vi "BatterySimulator.vi"() -> ()   [LabVIEW 2015]
panel:
  out "Waveform Graph 2":i32[](graph)
  out "Waveform Graph":dbl[](graph)
  out "exp(x)":fxp<+/-,64,32>
  out "x*y":dbl
  out "x/y":dbl
  out "Is":dbl
  out "Is  factor":dbl
  out "x-y":dbl
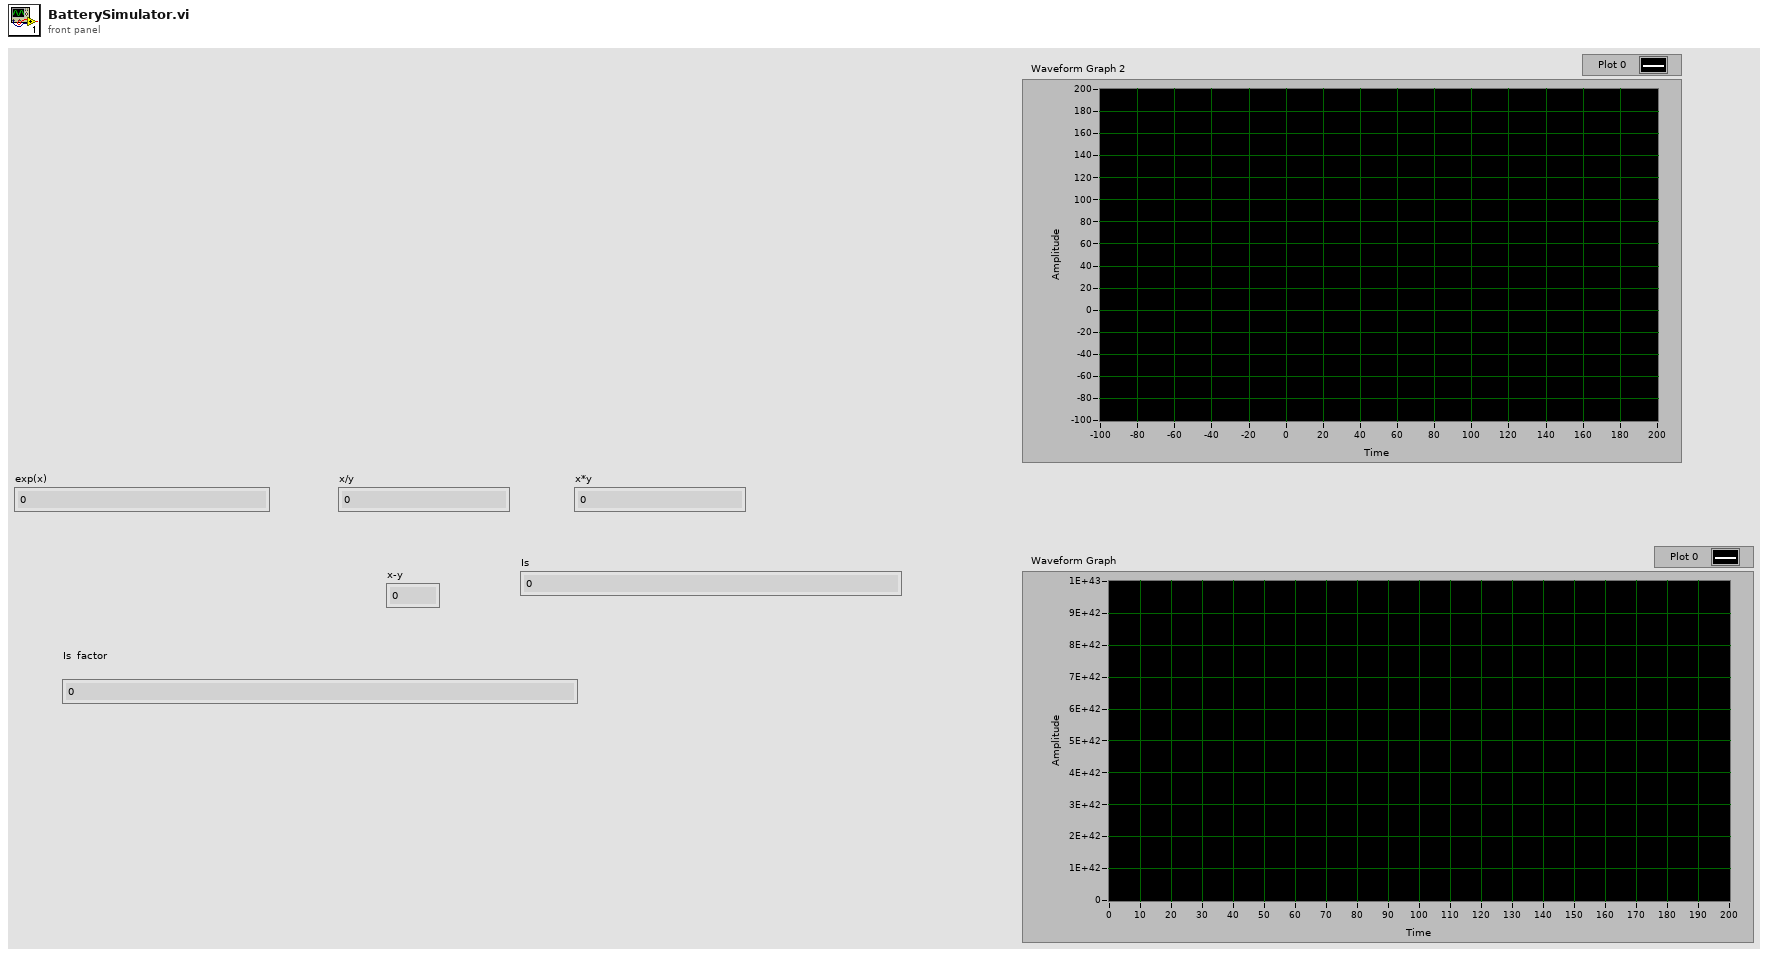
[diagram p1: front panel]
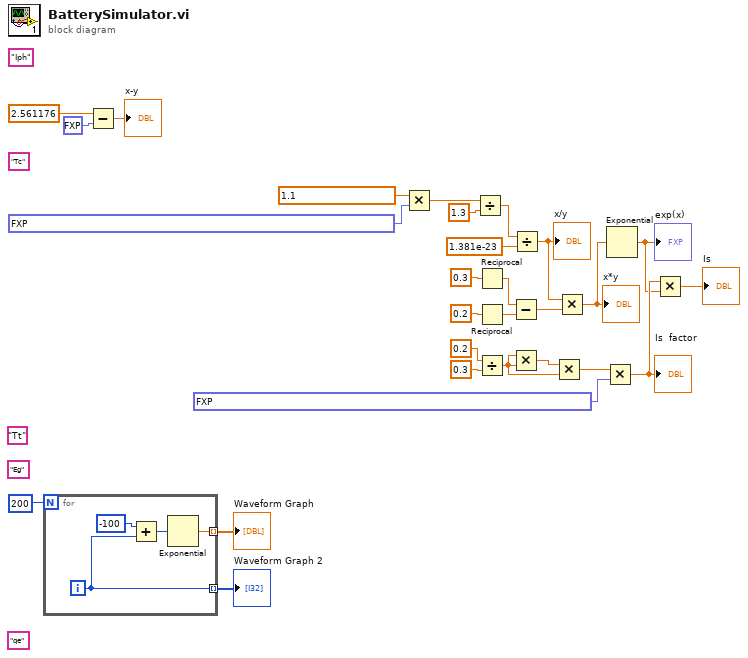
[diagram p0: block diagram]
diagram:
  (unwired) "Eg"
  (unwired) "qe"
  (unwired) "Tt"
  (unwired) "Tc"
  (unwired) "Iph"
  n1 = for {
    N: 200 -> [_]
    tunnel: [w30] -> w2 mode=indexing
    tunnel: [w29] -> w1 mode=indexing
    i -> [w29]
    n2 = Add(x=-100, y=w29) -> (x+y=w32:i32)
    n3 = Exponential(1:w32) -> (0:w30:dbl)
  }
  "Waveform Graph" <- w2
  "Waveform Graph 2" <- w1
  n4 = Subtract(x=2.561176, y=fxp<+,1,1> 0.0) -> (x-y=→"x-y":dbl)
  n5 = Multiply(x=1.1, y=fxp<+,15,-62> 1.6020172359436998e-19) -> (x*y=w14:dbl)
  n6 = Divide(x=w14, y=1.3) -> (x/y=w12:dbl)
  n7 = Reciprocal(x=0.3) -> (1/x=w8:dbl)
  n8 = Reciprocal(x=0.2) -> (1/x=w7:dbl)
  n9 = Divide(x=0.2, y=0.3) -> (x/y=w21:dbl)
  n10 = Subtract(x=w8, y=w7) -> (x-y=w5:dbl)
  n11 = Multiply(x=w21, y=w21) -> (x*y=w22:dbl)
  n12 = Divide(x=w12, y=1.381e-23) -> (x/y=w10:dbl)
  "x/y" <- w10
  n13 = Multiply(x=w22, y=w21) -> (x*y=w20:dbl)
  n14 = Multiply(x=w10, y=w5) -> (x*y=w4:dbl)
  "x*y" <- w4
  n15 = Multiply(x=w20, y=fxp<+,64,-42> 1.7307099956446998e-13) -> (x*y=w19:dbl)
  "Is  factor" <- w19
  n16 = Exponential(1:w4) -> (0:w18:dbl)
  "exp(x)" <- w18
  n17 = Multiply(x=w19, y=w18) -> (x*y=→"Is":dbl)
